vi "PH_Sixpack.get Axis i Attribute.vi"(0 "VI in":refnum<vi>, 2 "Axis":i32, 5 "error in":errorcluster) -> (13 "Axis Base Class Attributes":T1={"Settings"={"Sign change"=FALSE, "Width"=0.0, "Calibration"=0.0, "Unit"="", "Motor Type"=enum."Unspecific", "Unit Width"="", "Unit CF"=""}, "Endswitch?"=FALSE, "DIM Service IDs"={"Settings"=-1, "Information"=-1}, "Activity"=enum."No Information", "Configured?"=FALSE, "Position"={"Current"=0, "Target"=0}, "Position to set"={"New?"=FALSE, "Wanted"=0}, "Stop?"=FALSE, "Reset?"=FALSE, "Move?"=FALSE, "Nothing connected?"=FALSE}, 14 "VI out":refnum<vi>, 15 "HANDLE":i32, 16 "SixPack ID(0)":u16, 17 "Axis found?":bool, 18 "Axis Attributes":T6={"Config"={"VmaxAmax"={"VMax(511)"=0, "AMax(128)"=0}, "I max (50%)"=0.0, "VStartVminDivi"={"VStart(5)"=250, "Vmin(4)"=200, "Div i (2)"=enum."2"}, "Ref Search Parameter"={"VRefMax(100)"=100, "DebouncingTime (22ms)"=34}, "Stopswitch Limits"={"MinLeft(0)"=150, "MaxRight(1023)"=900}, "Axis Parameter"={"Poslimit (6400)"=150, "P5 Bits"={"MT_PI"=FALSE, "MT_ROTARY"=FALSE, "MT_AUTONULLCMD"=FALSE, "MT_TESTNULL"=FALSE, "MT_NULLLEFT"=FALSE, "MT_NULLCENTRE"=FALSE, "MT_STOPNULL"=FALSE, "MT_FILTERSWITCH"=FALSE}, "P6 Bits"={"MT_OPTIMIZEWAY"=FALSE, "MT_FASTREF"=FALSE, "MT_MECHREF"=FALSE, "MT_DELAYTESTNULL"=FALSE, "MT_STOPSOFT"=FALSE, "MT_STOPNOREF"=FALSE, "MT_NULLPOSITIVE"=FALSE, "MUT_STOPFULSTEPS"=FALSE}}, "I Control"={"PowerDownDelay (500)"=6400, "PowerDown (0%)"=enum."50%", "Standing (50%)"=enum."100%", "Running (75%)"=enum."100%", "Accelerating (100%)"=enum."100%"}}, "To set?"={"VmaxAmax"=FALSE, "I max"=FALSE, "VStartVminDivi"=FALSE, "Ref Search Parameter"=FALSE, "Stopswitch Limits"=FALSE, "Axis Parameter"=FALSE, "I Control"=FALSE}} {"Config"."Axis Parameter"."Poslimit (6400)" step=1; "Config"."Ref Search Parameter"."DebouncingTime (22ms)" format="%.0x"; "Config"."I max (50%)" min=0.0 max=100.0}, 19 "error out":errorcluster)   [LabVIEW 2014, in "PH_Sixpack.lvlib"]
uses:
  PH_Sixpack.lvlib
  PH_Sixpack.Axis Cluster.ctl
  PH_Sixpack.Axis Configuration.ctl
  instr.lib/Sixpack/PackDLL/VmaxAmax.ctl
  instr.lib/Sixpack/PackDLL/PeakCurrent.ctl
  instr.lib/Sixpack/PackDLL/VStartVmin.ctl
  instr.lib/Sixpack/PackDLL/Ref Search Parameter.ctl
  instr.lib/Sixpack/PackDLL/Stopswitch Limits.ctl
  instr.lib/Sixpack/PackDLL/Motor Parameter.ctl
  instr.lib/Sixpack/PackDLL/MotorParameter_P5.ctl
  instr.lib/Sixpack/PackDLL/MotorParameter_P6.ctl
  instr.lib/Sixpack/PackDLL/Current Control.ctl
  instr.lib/Sixpack/PackDLL/Current.ctl
  PH_Basics/PH_Stepmotor_BaseClass/PH_Stepmotor_BaseClass.Axis Attributes.ctl
  PH_Basics/PH_Stepmotor_BaseClass/PH_Stepmotor_BaseClass.Axis Settings.ctl
  PH_Basics/PH_Stepmotor_BaseClass/PH_Stepmotor_BaseClass.Motor Type.ctl
  PH_Basics/PH_Stepmotor_BaseClass/PH_Stepmotor_BaseClass.Axis DIM Service IDs.ctl
  PH_Basics/PH_Stepmotor_BaseClass/PH_Stepmotor_BaseClass.Axis Activity.ctl
  instr.lib/Sixpack/Sixpack - Driver.lvlib
  PH_Basics/PH_Stepmotor_BaseClass/PH_Stepmotor_BaseClass.lvlib
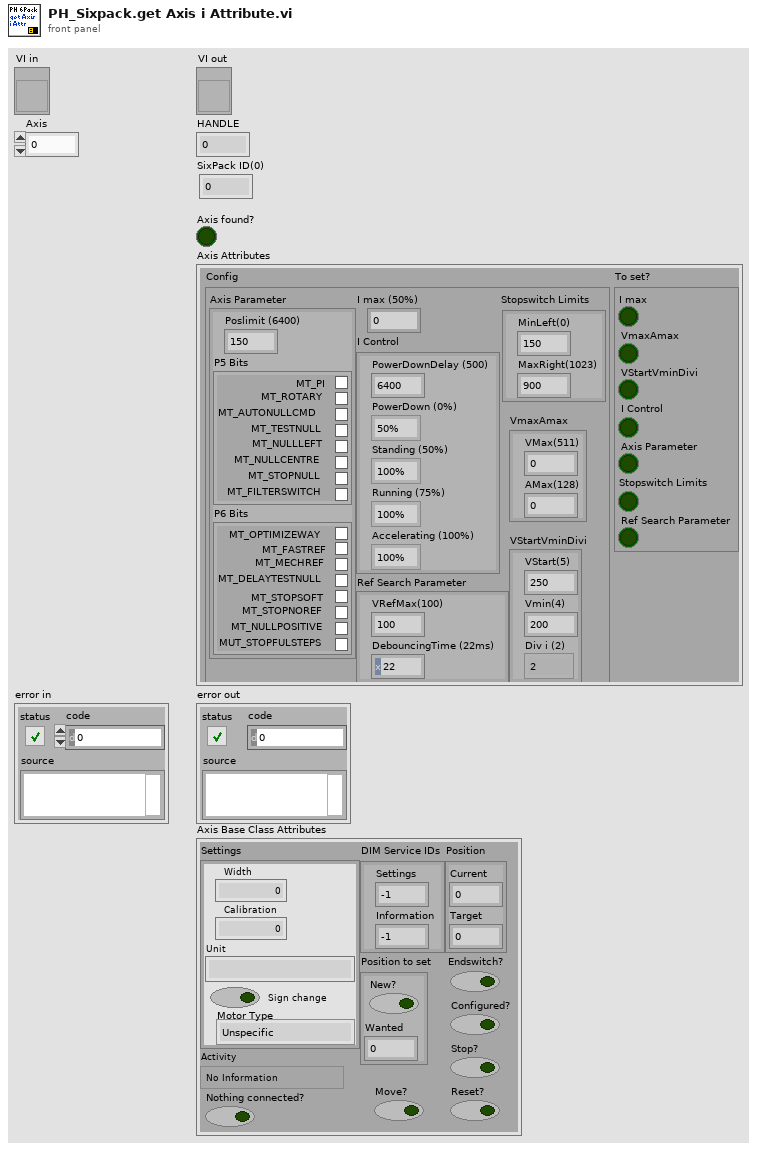
[diagram p1: front panel]
types:
  T1 = typedef "PH_Stepmotor_BaseClass.lvlib/PH_Stepmotor_BaseClass.Axis Attributes.ctl" = cluster{"Settings":T2, "Endswitch?":bool, "DIM Service IDs":T4, "Activity":T5, "Configured?":bool, "Position":cluster{"Current":i32, "Target":i32}, "Position to set":cluster{"New?":bool, "Wanted":i32}, "Stop?":bool, "Reset?":bool, "Move?":bool, "Nothing connected?":bool}
  T2 = typedef "PH_Stepmotor_BaseClass.lvlib/PH_Stepmotor_BaseClass.Axis Settings.ctl" = cluster{"Sign change":bool, "Width":dbl, "Calibration":dbl, "Unit":string, "Motor Type":T3, "Unit Width":string, "Unit CF":string}
  T3 = typedef "PH_Stepmotor_BaseClass.lvlib/PH_Stepmotor_BaseClass.Motor Type.ctl" = enum16{"Unspecific", "OWIS 49.120.2633", "OWIS 49.060.1033", "OWIS 43.040.2558", "Diamond Motion 2200 series", "OWIS 49.120.266B.MV6", "Calorimeter", "Linear Stage 1", "MICOS VT-80", "MICOS VT-80 S", "Standa Rotstage nt0.95A", "PUF RA 320.200", "PUF RA 800.200", "PUF RA 800.400", "PUF RA 400.50", "1324.nn.800.50", "1324.n9c.800.50", "1324.nn.320.200", "1324.nn.400.200", "1324.nn.800.200", "1324.nn.400.50", "1324.8c9c.800.50", "1324.8c9c.400.200"}
  T4 = typedef "PH_Stepmotor_BaseClass.lvlib/PH_Stepmotor_BaseClass.Axis DIM Service IDs.ctl" = cluster{"Settings":i32, "Information":i32}
  T5 = typedef "PH_Stepmotor_BaseClass.lvlib/PH_Stepmotor_BaseClass.Axis Activity.ctl" = enum16{"No Information", "stopped", "running", "Failure", "Alarm", "stopped at backward ES", "stopped at foreward ES"}
  T6 = typedef "PH_Sixpack.lvlib/PH_Sixpack.Axis Cluster.ctl" = cluster{"Config":T7, "To set?":cluster{"VmaxAmax":bool, "I max":bool, "VStartVminDivi":bool, "Ref Search Parameter":bool, "Stopswitch Limits":bool, "Axis Parameter":bool, "I Control":bool}}
  T7 = typedef "PH_Sixpack.lvlib/PH_Sixpack.Axis Configuration.ctl" = cluster{"VmaxAmax":T8, "I max (50%)":T9, "VStartVminDivi":T10, "Ref Search Parameter":T11, "Stopswitch Limits":T12, "Axis Parameter":T13, "I Control":T16}
  T8 = typedef "Sixpack - Driver.lvlib/VmaxAmax.ctl" = cluster{"VMax(511)":u16, "AMax(128)":u16}
  T9 = typedef "Sixpack - Driver.lvlib/PeakCurrent.ctl" = dbl
  T10 = typedef "Sixpack - Driver.lvlib/VStartVmin.ctl" = cluster{"VStart(5)":u16, "Vmin(4)":u16, "Div i (2)":enum8{"0", "1", "2", "3"}}
  T11 = typedef "Sixpack - Driver.lvlib/Ref Search Parameter.ctl" = cluster{"VRefMax(100)":u16, "DebouncingTime (22ms)":u8}
  T12 = typedef "Sixpack - Driver.lvlib/Stopswitch Limits.ctl" = cluster{"MinLeft(0)":u16, "MaxRight(1023)":u16}
  T13 = typedef "Sixpack - Driver.lvlib/Motor Parameter.ctl" = cluster{"Poslimit (6400)":u32, "P5 Bits":T14, "P6 Bits":T15}
  T14 = typedef "Sixpack - Driver.lvlib/MotorParameter_P5.ctl" = cluster{"MT_PI":bool, "MT_ROTARY":bool, "MT_AUTONULLCMD":bool, "MT_TESTNULL":bool, "MT_NULLLEFT":bool, "MT_NULLCENTRE":bool, "MT_STOPNULL":bool, "MT_FILTERSWITCH":bool}
  T15 = typedef "Sixpack - Driver.lvlib/MotorParameter_P6.ctl" = cluster{"MT_OPTIMIZEWAY":bool, "MT_FASTREF":bool, "MT_MECHREF":bool, "MT_DELAYTESTNULL":bool, "MT_STOPSOFT":bool, "MT_STOPNOREF":bool, "MT_NULLPOSITIVE":bool, "MUT_STOPFULSTEPS":bool}
  T16 = typedef "Sixpack - Driver.lvlib/Current Control.ctl" = cluster{"PowerDownDelay (500)":u16, "PowerDown (0%)":T17, "Standing (50%)":T17, "Running (75%)":T17, "Accelerating (100%)":T17}
  T17 = typedef "Sixpack - Driver.lvlib/Current.ctl" = enum8{"100%", "75%", "50%", "38%", "25%", "19%", "13%", "9%", "0%"}
  T18 = typedef "PH_Sixpack.lvlib/PH_Sixpack.i attribute.ctl" = cluster{"Information":cluster{"SixPack ID(0)":u16, "BaudRate(19200)":u16, "COM Port":enum32{"COM1", "COM2", "COM3", "COM4", "COM5", "COM6", "COM7", "COM8", "COM9"}, "HANDLE":i32}, "Serial Number":dbl, "Firmwareversion":dbl, "Axes":T6[], "Status":T19, "Axis to do a RefSearch":i32, "GUI Refs":cluster{"Information":refnum<vi>, "Serial Number":refnum<vi>, "Firmwareversion":refnum<vi>, "Status":refnum<vi>, "Axis to do a RefSearch":refnum<vi>, "Axes Configuration (Sixpack)":refnum<vi>, "Inputs":refnum<vi>, "PeriodicInterval [ms]":refnum<vi>}, "Constructor finished":bool, "Ignore Error":bool}
  T19 = typedef "PH_Sixpack.lvlib/PH_Sixpack.Status.ctl" = enum32{"None", "Init", "Configure", "configured", "Close", "closed"}
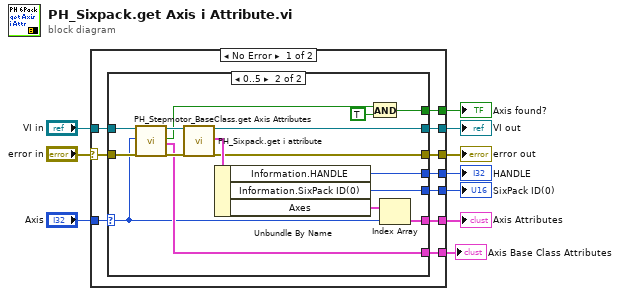
[diagram p0: block diagram]
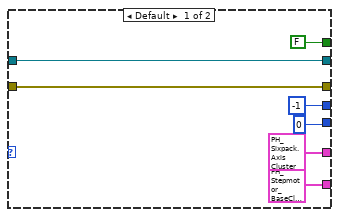
[diagram p2: hidden frame]
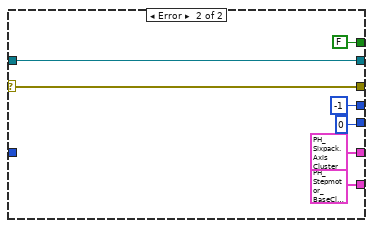
[diagram p3: hidden frame]
diagram:
  n1 = case shown="No Error" "error in" {
    selector: "error in" -> [w15 w49]
    tunnel: [w20 T6 {"Config"={"VmaxAmax"={"VMax(511)"=128, "AMax(128)"=300}, "I max (50%)"=200.0, "VStartVminDivi"={"VStart(5)"=2, "Vmin(4)"=250, "Div i (2)"=enum."2"}, "Ref Search Parameter"={"VRefMax(100)"=100, "DebouncingTime (22ms)"=34}, "Stopswitch Limits"={"MinLeft(0)"=150, "MaxRight(1023)"=900}, "Axis Parameter"={"Poslimit (6400)"=128, "P5 Bits"={"MT_PI"=FALSE, "MT_ROTARY"=FALSE, "MT_AUTONULLCMD"=FALSE, "MT_TESTNULL"=FALSE, "MT_NULLLEFT"=FALSE, "MT_NULLCENTRE"=FALSE, "MT_STOPNULL"=FALSE, "MT_FILTERSWITCH"=FALSE}, "P6 Bits"={"MT_OPTIMIZEWAY"=FALSE, "MT_FASTREF"=FALSE, "MT_MECHREF"=FALSE, "MT_DELAYTESTNULL"=FALSE, "MT_STOPSOFT"=FALSE, "MT_STOPNOREF"=FALSE, "MT_NULLPOSITIVE"=FALSE, "MUT_STOPFULSTEPS"=FALSE}}, "I Control"={"PowerDownDelay (500)"=0, "PowerDown (0%)"=enum."100%", "Standing (50%)"=enum."100%", "Running (75%)"=enum."100%", "Accelerating (100%)"=enum."100%"}}, "To set?"={"VmaxAmax"=FALSE, "I max"=FALSE, "VStartVminDivi"=FALSE, "Ref Search Parameter"=FALSE, "Stopswitch Limits"=FALSE, "Axis Parameter"=FALSE, "I Control"=FALSE}} ("motor")] -> w10
    tunnel: [w19 w50] -> w9
    tunnel: "VI in" -> [w18 w50]
    tunnel: [w17 w49] -> w7
    tunnel: "Axis" -> [w16 _]
    tunnel: [w14 FALSE] -> w4
    tunnel: [w13 u16 0 ("SixPack ID(0)")] -> w3
    tunnel: [w12 -1 ("HANDLE")] -> w2
    tunnel: [w11 T1 {"Settings"={"Sign change"=FALSE, "Width"=0.0, "Calibration"=0.0, "Unit"="", "Motor Type"=enum."Unspecific", "Unit Width"="", "Unit CF"=""}, "Endswitch?"=FALSE, "DIM Service IDs"={"Settings"=-1, "Information"=-1}, "Activity"=enum."No Information", "Configured?"=FALSE, "Position"={"Current"=0, "Target"=0}, "Position to set"={"New?"=FALSE, "Wanted"=0}, "Stop?"=FALSE, "Reset?"=FALSE, "Move?"=FALSE, "Nothing connected?"=FALSE} ("motor")] -> w1
    frame No Error {
      n2 = case shown="0..5" w16 {
        selector: w16 -> [_ w30]
        tunnel: [T6 {"Config"={"VmaxAmax"={"VMax(511)"=128, "AMax(128)"=300}, "I max (50%)"=200.0, "VStartVminDivi"={"VStart(5)"=2, "Vmin(4)"=250, "Div i (2)"=enum."2"}, "Ref Search Parameter"={"VRefMax(100)"=100, "DebouncingTime (22ms)"=34}, "Stopswitch Limits"={"MinLeft(0)"=150, "MaxRight(1023)"=900}, "Axis Parameter"={"Poslimit (6400)"=128, "P5 Bits"={"MT_PI"=FALSE, "MT_ROTARY"=FALSE, "MT_AUTONULLCMD"=FALSE, "MT_TESTNULL"=FALSE, "MT_NULLLEFT"=FALSE, "MT_NULLCENTRE"=FALSE, "MT_STOPNULL"=FALSE, "MT_FILTERSWITCH"=FALSE}, "P6 Bits"={"MT_OPTIMIZEWAY"=FALSE, "MT_FASTREF"=FALSE, "MT_MECHREF"=FALSE, "MT_DELAYTESTNULL"=FALSE, "MT_STOPSOFT"=FALSE, "MT_STOPNOREF"=FALSE, "MT_NULLPOSITIVE"=FALSE, "MUT_STOPFULSTEPS"=FALSE}}, "I Control"={"PowerDownDelay (500)"=0, "PowerDown (0%)"=enum."100%", "Standing (50%)"=enum."100%", "Running (75%)"=enum."100%", "Accelerating (100%)"=enum."100%"}}, "To set?"={"VmaxAmax"=FALSE, "I max"=FALSE, "VStartVminDivi"=FALSE, "Ref Search Parameter"=FALSE, "Stopswitch Limits"=FALSE, "Axis Parameter"=FALSE, "I Control"=FALSE}} ("motor") w43] -> w20
        tunnel: [w27 w40] -> w19
        tunnel: w18 -> [w27 w35]
        tunnel: [w26 w39] -> w17
        tunnel: w15 -> [w26 w33]
        tunnel: [FALSE w29] -> w14
        tunnel: [u16 0 ("SixPack ID(0)") w37] -> w13
        tunnel: [-1 ("HANDLE") w36] -> w12
        tunnel: [T1 {"Settings"={"Sign change"=FALSE, "Width"=0.0, "Calibration"=0.0, "Unit"="", "Motor Type"=enum."Unspecific", "Unit Width"="", "Unit CF"=""}, "Endswitch?"=FALSE, "DIM Service IDs"={"Settings"=-1, "Information"=-1}, "Activity"=enum."No Information", "Configured?"=FALSE, "Position"={"Current"=0, "Target"=0}, "Position to set"={"New?"=FALSE, "Wanted"=0}, "Stop?"=FALSE, "Reset?"=FALSE, "Move?"=FALSE, "Nothing connected?"=FALSE} ("motor") w31] -> w11
        frame Default {
        }
        frame 0..5 {
          n3 = call "PH_Stepmotor_BaseClass.get Axis Attributes.vi"("VI in"=w35, "Axis"=w30, "error in (no error)"=w33) -> ("VI out"=w34:refnum<vi>, "Axis found?"=w28:bool, "Axis Attributes"=w31:T1, "error out"=w32:errorcluster)  [unwired: 13 in]
          n4 = call "PH_Sixpack.get i attribute.vi"("i ref in"=w34, "error in (no error)"=w32) -> ("i ref out"=w40:refnum<vi>, "i attribute"=w41:T18, "error out"=w39:errorcluster)  [unwired: 15 in]
          n5 = Unbundle By Name(w41) -> ("Information.HANDLE"=w36:i32, "Information.SixPack ID(0)"=w37:u16, "Axes"=w42:T6[])
          n6 = And(x=w28, y=TRUE) -> (x .and. y?=w29:bool)
          n7 = Index Array(array=w42, index=w30) -> (element=w43:T6)
        }
      }
    }
    frame Error {
    }
  }
  "Axis Attributes" <- w10
  "VI out" <- w9
  "error out" <- w7
  "Axis found?" <- w4
  "SixPack ID(0)" <- w3
  "HANDLE" <- w2
  "Axis Base Class Attributes" <- w1
